vi "FTW-Bootstrapper-Initialize.vi"(0 "Uninitialized FTW Bootstrapper":refnum<class "FTW-Actor-Bootstrapper.lvclass">, 5 "Actor VI Filepath":path, 7 "Actor Configuration":string, 11 "error in":errorcluster) -> (4 "FTW Bootstrapper":refnum<class "FTW-Actor-Bootstrapper.lvclass">, 15 "error out":errorcluster)   [LabVIEW 2012, in "FTW-Actor-Bootstrapper.lvclass"]
uses:
  FTW-Actor-Bootstrapper.lvclass
  Context/FTW-Actor-Context.lvclass
  Reference/FTW-ActorReference.lvclass
panel:
  # "Inputs"
  # "Outputs"
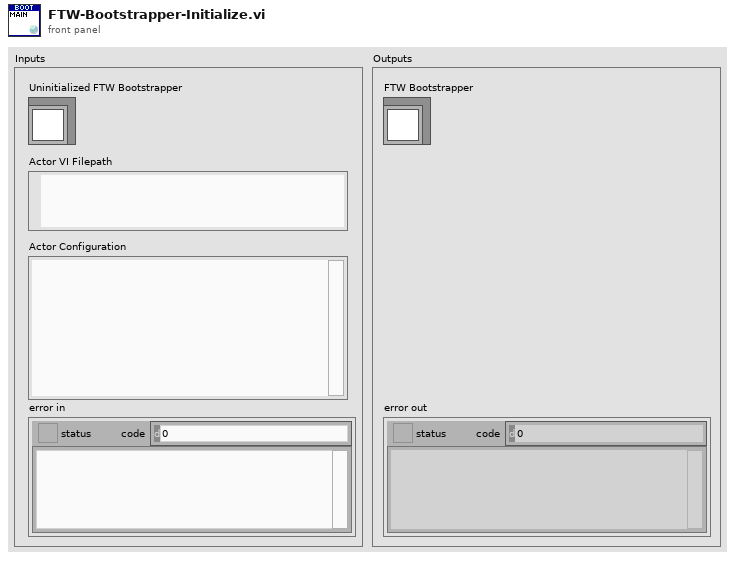
[diagram p1: front panel]
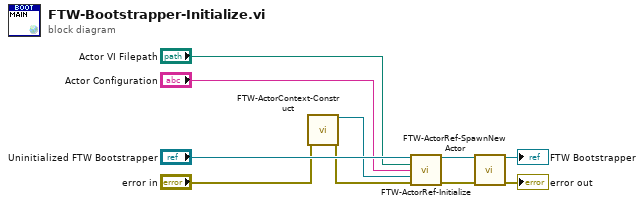
[diagram p0: block diagram]
diagram:
  n1 = call "FTW-ActorContext-Construct.vi"("error in"="error in") -> ("FTW Actor Context"=w5:refnum<class "FTW-Actor-Context.lvclass">, "error out"=w4:errorcluster)  [unwired: 13 in]
  n2 = call "FTW-ActorRef-Initialize.vi"("FTW Actor Reference"="Uninitialized FTW Bootstrapper", "Actor VI Filepath"="Actor VI Filepath", "Actor Configuration"="Actor Configuration", "Actor Context"=w5, "error in"=w4) -> ("FTW Actor Reference out"=w6:refnum<class "FTW-Actor-Bootstrapper.lvclass">, "error out"=w3:errorcluster)  [unwired: 9 in]
  n3 = call-dynamic "FTW-ActorRef-SpawnNewActor.vi"("Actor Ref Prototype"=w6, "error in"=w3) -> ("Actor Reference"=→"FTW Bootstrapper":refnum<class "FTW-Actor-Bootstrapper.lvclass">, "error out"=→"error out":errorcluster)  [unwired: 12 in]
